vi "CRYCal Perceptual Rub&buzz.vi"(6 "Fs":dbl=44100.0, 8 "TSR params":T2={"FSamp"=44100.0, "FStart"=20.0, "FStop"=20000.0, "NOffset"=0.0, "MStop"=132741.0, "MStart"=441.0, "NHarm"=19152.386651933408, "Tsamp"=2.2675736961451248e-05, "Amplit"=1.0, "Sweep Time"=1.0} {"Sweep Time" format="%.2f"; "Amplit" format="%.2f"; "FStop" format="%.2f"; "FStart" format="%.2f"; "FSamp" format="%.2f"; "Tsamp" format="%.2f"; "NHarm" format="%.2f"; "MStart" format="%.2f"; "MStop" format="%.2f"; "NOffset" format="%.2f"}, 9 "Harmonic Infor":T1={"Cycles"=[200.0, 190.0, 180.0, 170.0, 160.0, 150.0, 140.0, 132.0, 125.0, 118.0, 112.0, 106.0, 100.0, 95.0, 90.0, 85.0, 80.0, 75.0, 71.0, 67.0, 63.0, 60.0, 56.0, 53.0, 50.0, 48.0, 45.0, 43.0, 40.0, 38.0, 36.0, 34.0, 32.0, 30.0, 28.0, 27.0, 25.0, 24.0, 23.0, 22.0, 20.0, 19.0, 18.0, 17.0, 16.0, 15.0, 14.0, 14.0, 13.0, 12.0, 12.0, 11.0, 10.0, 10.0, 9.0, 9.0, 8.0, 8.0, 8.0, 7.0, 7.0, 6.0, 6.0, 6.0, 6.0, 6.0, 6.0, 6.0, 6.0, 6.0, 6.0, 6.0, 6.0, 6.0, 8.0, 8.0, 8.0, 8.0, 8.0, 8.0, 8.0, 8.0], "Frequency"=[20000.0, 19000.0, 18000.0, 17000.0, 16000.0, 15000.0, 14000.0, 13199.999809265137, 12500.0, 11800.000190734863, 11199.999809265137, 10600.000381469727, 10000.0, 9500.0, 9000.0, 8500.0, 8000.0, 7500.0, 7099.999904632568, 6699.999809265137, 6300.000190734863, 6000.0, 5599.999904632568, 5300.000190734863, 5000.0, 4750.0, 4500.0, 4250.0, 4000.0, 3750.0, 3549.999952316284, 3349.9999046325684, 3150.0000953674316, 3000.0, 2799.999952316284, 2650.0000953674316, 2500.0, 2359.999895095825, 2240.000009536743, 2119.999885559082, 2000.0, 1900.0, 1800.0, 1700.0, 1600.0, 1500.0, 1400.0, 1319.9999809265137, 1250.0, 1180.0000190734863, 1119.9999809265137, 1060.0000381469727, 1000.0, 950.0, 900.0, 850.0, 800.0, 750.0, 709.9999904632568, 669.9999809265137, 630.0000190734863, 600.0, 559.9999904632568, 530.0000190734863, 500.0, 475.0, 450.0, 425.0, 400.0, 375.0, 354.9999952316284, 334.99999046325684, 315.00000953674316, 300.0, 250.0, 200.0, 160.0, 125.0, 100.0, 80.0, 63.00000190734863, 50.0], "Amplitude"=[0.5, 0.5, 0.5, 0.5, 0.5, 0.5, 0.5, 0.5, 0.5, 0.5, 0.5, 0.5, 0.5, 0.5, 0.5, 0.5, 0.5, 0.5, 0.5, 0.5, 0.5, 0.5, 0.5, 0.5, 0.5, 0.5, 0.5, 0.5, 0.5, 0.5, 0.5, 0.5, 0.5, 0.5, 0.5, 0.5, 0.5, 0.5, 0.5, 0.5, 0.5, 0.5, 0.5, 0.5, 0.5, 0.5, 0.5, 0.5, 0.5, 0.5, 0.5, 0.5, 0.5, 0.5, 0.5, 0.5, 0.5, 0.5, 0.5, 0.5, 0.5, 0.5, 0.5, 0.5, 0.5, 0.5, 0.5, 0.5, 0.5, 0.5, 0.5, 0.5, 0.5, 0.5, 0.5, 0.5, 0.5, 0.5, 0.5, 0.5, 0.5, 0.5], "samples"=[441, 441, 441, 441, 441, 441, 441, 441, 441, 441, 441, 441, 441, 441, 441, 441, 441, 441, 441, 441, 441, 441, 441, 441, 441, 446, 441, 446, 441, 447, 447, 447, 448, 441, 441, 450, 441, 448, 453, 458, 441, 441, 441, 441, 441, 441, 441, 467, 459, 448, 473, 458, 441, 464, 441, 467, 441, 470, 497, 461, 490, 441, 472, 499, 530, 557, 588, 622, 662, 705, 746, 790, 840, 882, 1411, 1764, 2205, 2823, 3528, 4410, 5600, 7055], "Fs"=44100.0, "window"=7, "discard cycles"=1.0} {"discard cycles" min=1.0}, 10 "Response":dbl[](array[numeric]) format="%.2f", 11 "Stimulus":dbl[](array[numeric])=array[132785 elements] format="%.2f") -> (2 "EHS + NL":dbl[](array[numeric]), 3 "Frequency":dbl[](array[numeric]))   [LabVIEW 2013]
panel:
  out "samples":i32[](array[numeric])
  out "Frequency 2":dbl[](array[numeric])
  out "Cycles":dbl[](array[numeric])
  out "Response Wave":waveform(dbl)(graph)
  out "Stimulus Wave":waveform(dbl)(graph)
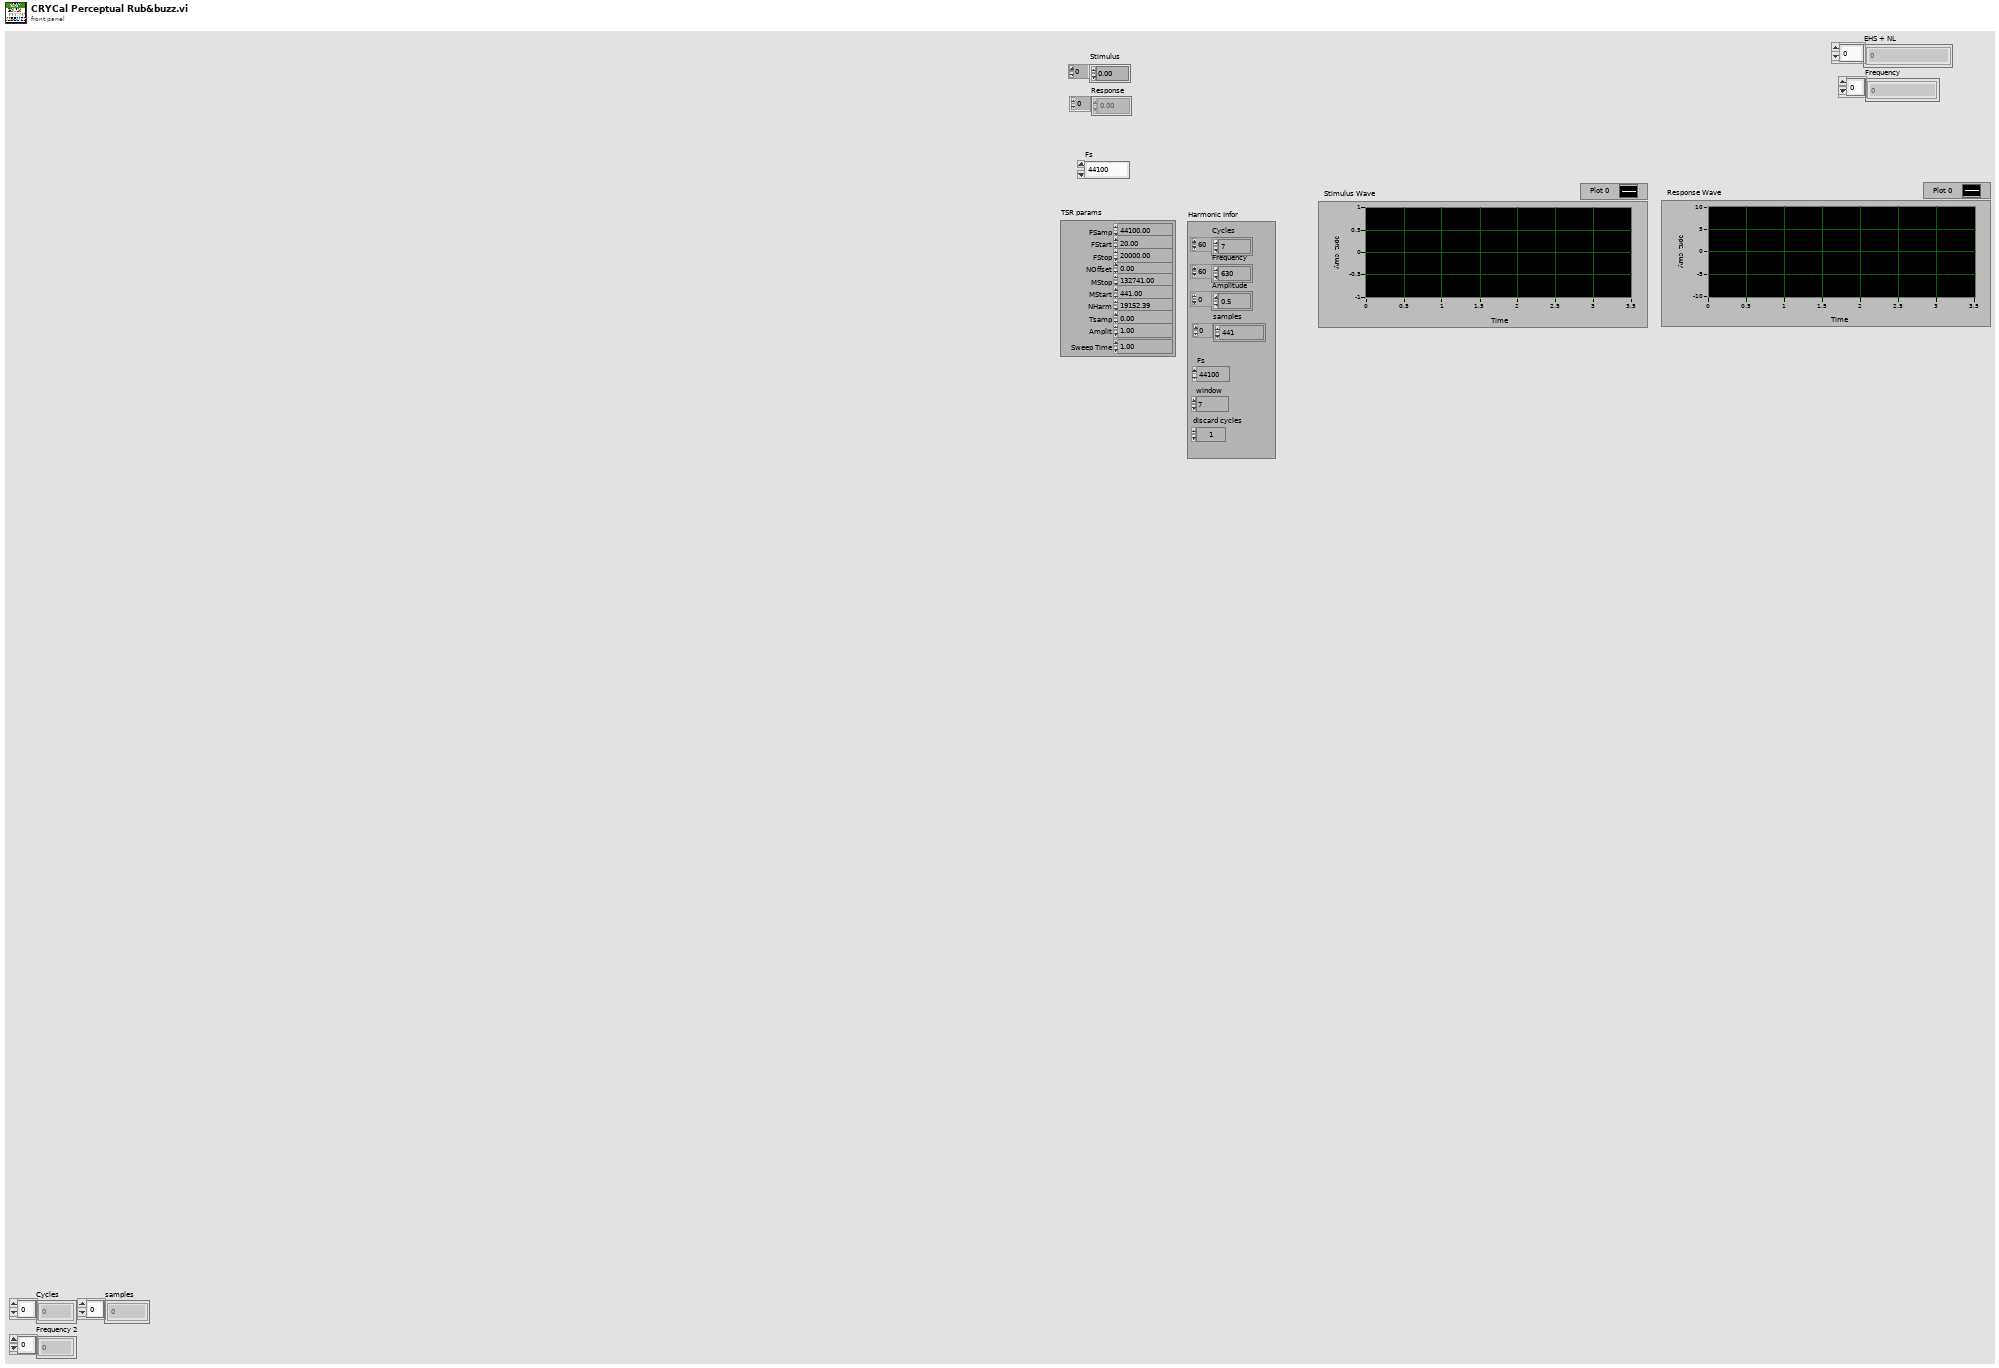
[diagram p1: front panel]
types:
  T1 = cluster{"Cycles":dbl[], "Frequency":dbl[], "Amplitude":dbl[], "samples":i32[], "Fs":dbl, "window":u16, "discard cycles":dbl}
  T2 = cluster{"FSamp":dbl, "FStart":dbl, "FStop":dbl, "NOffset":dbl, "MStop":dbl, "MStart":dbl, "NHarm":dbl, "Tsamp":dbl, "Amplit":dbl, "Sweep Time":dbl}
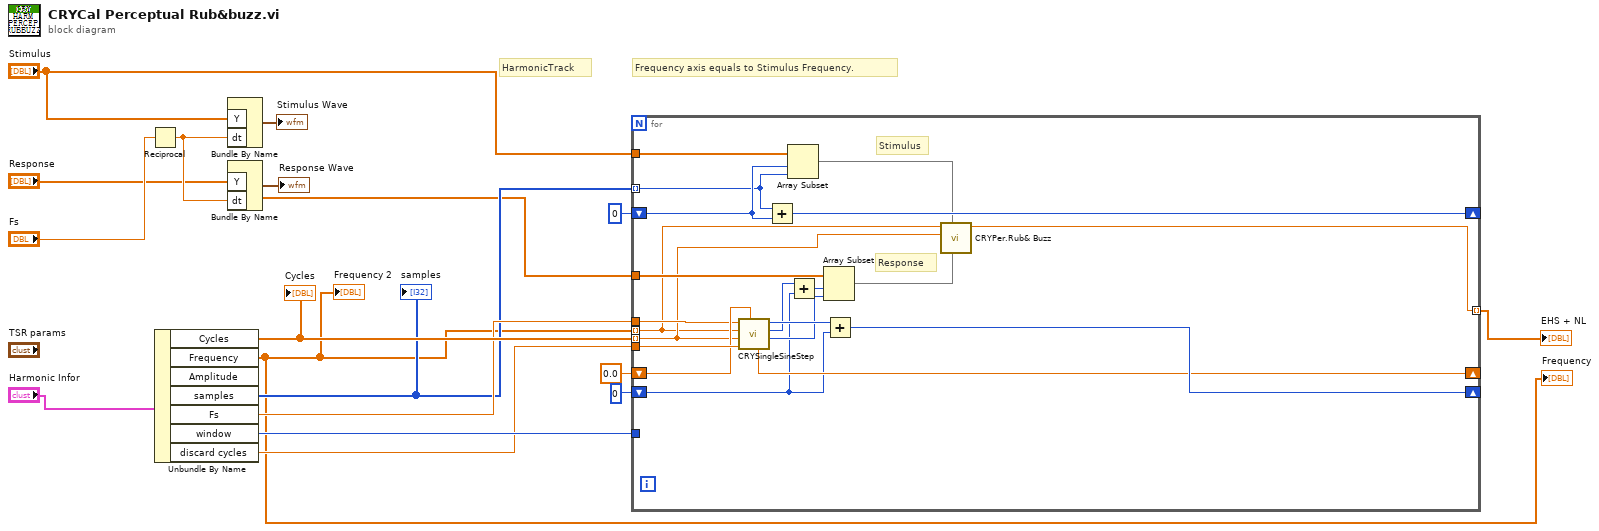
[diagram p0: block diagram]
diagram:
  # "Frequency axis equals to Stimulus Frequency."
  # "HarmonicTrack"
  n1 = Reciprocal(x="Fs") -> (1/x=w17:dbl)
  n2 = Unbundle By Name("Harmonic Infor") -> ("Cycles"=w13:dbl[], "Frequency"=w2:dbl[], "samples"=w9:i32[], "Fs"=w10:dbl, "window"=w12:u16, "discard cycles"=w11:dbl)  [unwired: 1 out]
  "Cycles" <- w13
  "Frequency 2" <- w2
  "samples" <- w9
  "Frequency" <- w2
  n3 = Bundle By Name("Y"="Stimulus", "dt"=w17) -> (→"Stimulus Wave":waveform(dbl))  [unwired: 1 in]
  n4 = Bundle By Name("Y"="Response", "dt"=w17) -> (→"Response Wave":waveform(dbl))  [unwired: 1 in]
  n5 = for {
    tunnel: w10 -> [w29]
    shift-right: [w37] -> _
    shift-left: 0 -> [w24]
    tunnel: "Response" -> [w33]
    tunnel: w13 -> [w20] mode=indexing
    tunnel: w2 -> [w19] mode=indexing
    tunnel: w11 -> [w36]
    shift-right: [w34] -> _
    shift-left: 0.0 -> [w35]
    tunnel: w12 -> [_]
    tunnel: [w18] -> w1 mode=indexing
    tunnel: "Stimulus" -> [w31]
    tunnel: w9 -> [w27] mode=indexing
    shift-right: [w30] -> _
    shift-left: 0 -> [w28]
    # "Response"
    # "Stimulus"
    n6 = call "CRYSingleSineStep.vi"("Fs"=w29, "Freq"=w19, "Cycles per freq"=w20, "Cycles discarded"=w36, "StartPhase"=w35) -> ("StopPhase"=w34:dbl, "TotalSamples"=w32:i32, "DiscardSamples"=w23:i32, "ExtractSamples"=w25:i32)  [unwired: 2 out]
    n7 = Add(x=w27, y=w28) -> (x+y=w30:i32)
    n8 = Array Subset(array=w31, index=w28, length=w27) -> (w21:dbl[])
    n9 = Add(x=w23, y=w24) -> (x+y=w26:i32)
    n10 = Array Subset(array=w33, index=w26, length=w25) -> (w22:dbl[])
    n11 = Add(x=w32, y=w24) -> (x+y=w37:i32)
    n12 = call "CRYPer.Rub& Buzz.vi"("response"=w22, "stimulus"=w21, "cycle"=w20, "frequency"=w19) -> ("out Y"=w18:dbl)  [unwired: 5 in]
  }
  "EHS + NL" <- w1
